vi "Open from file.vi"() -> (0 "Confign name":string, 3 "Cluster":T1)   [LabVIEW 2020]
uses:
  <vilib>/Utility/file.llb/Read Delimited Spreadsheet (string).vi
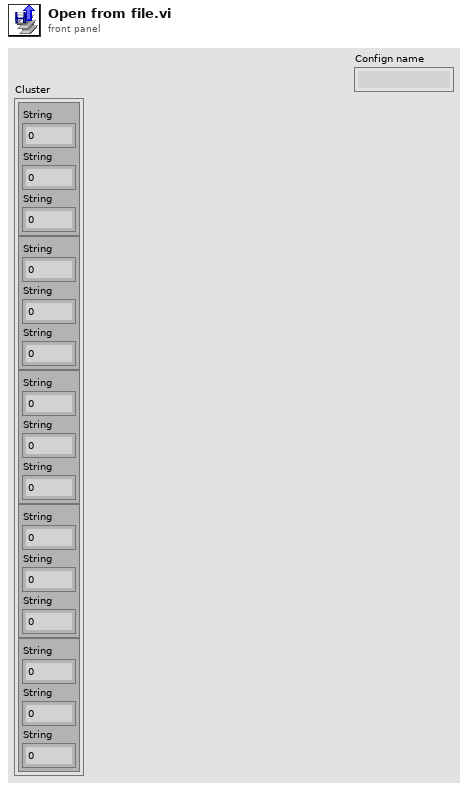
[diagram p1: front panel]
types:
  T1 = cluster{cluster{"String":i32, "String":i32, "String":i32}, cluster{"String":i32, "String":i32, "String":i32}, cluster{"String":i32, "String":i32, "String":i32}, cluster{"String":i32, "String":i32, "String":i32}, cluster{"String":i32, "String":i32, "String":i32}}
  T2 = cluster{"String":i32, "String":i32, "String":i32}
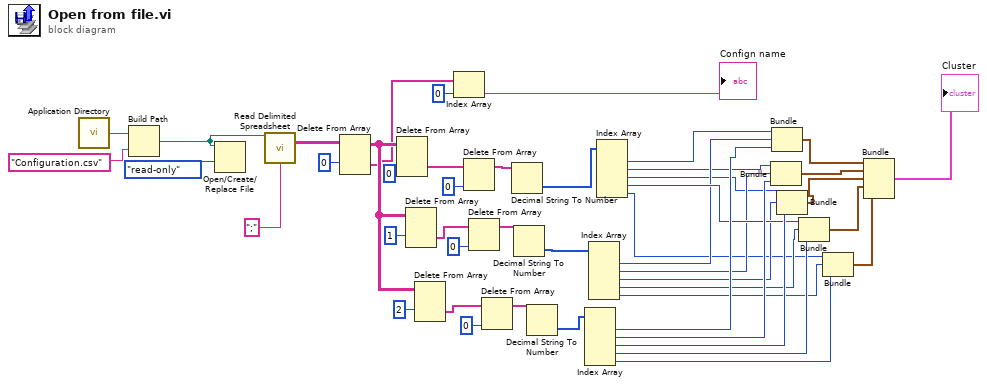
[diagram p0: block diagram]
diagram:
  n1 = call <vilib>:"Application Directory.vi"() -> ("Application Directory"=w6:path)
  n2 = Build Path(base path=w6, name or relative path="Configuration.csv") -> (appended path=w7:path)
  n3 = Open/Create/Replace File(file path (use dialog)=w7, access (0:read/write)=enum16{"read/write", "read-only", "write-only"}."read-only") -> ()  [unwired: 4 in, 3 out]
  n4 = call-poly <vilib>:"Read Delimited Spreadsheet.vi"("file path (dialog if empty)"=w7, "delimiter (\\t)"=";" ("delimiter (\\t)")) -> ("all rows"=w8:string[][])  [unwired: 8 in, 5 out]
  n5 = Delete From Array(array=w8, index (row)=0) -> (deleted portion=w3:string[], array with subset deleted=w31:string[][])  [unwired: 2 in]
  n6 = Delete From Array(array=w31, index (row)=0) -> (deleted portion=w19:string[])  [unwired: 2 in, 1 out]
  n7 = Delete From Array(array=w31, index (row)=1) -> (deleted portion=w23:string[])  [unwired: 2 in, 1 out]
  n8 = Delete From Array(array=w31, index (row)=2) -> (deleted portion=w35:string[])  [unwired: 2 in, 1 out]
  n9 = Index Array(array=w3, index=0) -> (element=→"Confign name":string)
  n10 = Delete From Array(array=w19, index=0) -> (array with subset deleted=w13:string[])  [unwired: 1 in, 1 out]
  n11 = Delete From Array(array=w23, index=0) -> (array with subset deleted=w22:string[])  [unwired: 1 in, 1 out]
  n12 = Delete From Array(array=w35, index=0) -> (array with subset deleted=w34:string[])  [unwired: 1 in, 1 out]
  n13 = Decimal String To Number(string=w13) -> (number=w14:i32[])  [unwired: 2 in, 1 out]
  n14 = Decimal String To Number(string=w22) -> (number=w24:i32[])  [unwired: 2 in, 1 out]
  n15 = Decimal String To Number(string=w34) -> (number=w36:i32[])  [unwired: 2 in, 1 out]
  n16 = Index Array(array=w36) -> (element #1=w37:i32, element #2=w38:i32, element #3=w39:i32, element #4=w40:i32, element #5=w41:i32)  [unwired: 5 in]
  n17 = Index Array(array=w24) -> (element #1=w25:i32, element #2=w26:i32, element #3=w27:i32, element #4=w29:i32, element #5=w30:i32)  [unwired: 5 in]
  n18 = Index Array(array=w14) -> (element #1=w15:i32, element #2=w16:i32, element #3=w17:i32, element #4=w28:i32, element #5=w18:i32)  [unwired: 5 in]
  n19 = Bundle("String"=w16, "String"=w26, "String"=w38) -> (w43:T2)  [unwired: 1 in]
  n20 = Bundle("String"=w15, "String"=w25, "String"=w37) -> (w42:T2)  [unwired: 1 in]
  n21 = Bundle("String"=w17, "String"=w27, "String"=w39) -> (w44:T2)  [unwired: 1 in]
  n22 = Bundle("String"=w28, "String"=w29, "String"=w40) -> (w45:T2)  [unwired: 1 in]
  n23 = Bundle("String"=w18, "String"=w30, "String"=w41) -> (w46:T2)  [unwired: 1 in]
  n24 = Bundle(w42, w43, w44, w45, w46) -> (→"Cluster":T1)  [unwired: 1 in]
